vi "Draw Legend Cluster.vi"(8 "error in (no error)":errorcluster, 9 "Plot Area Ref":refnum<vi>, 10 "Number Of Rows":i32, 11 "2D Feather.lvclass in":refnum<class "2D Feather.lvclass">) -> (0 "error out":errorcluster, 1 "Legend Cluster":T1(array[cluster]), 3 "2D Feather.lvclass out":refnum<class "2D Feather.lvclass">)   [LabVIEW 2017, in "2D Feather.lvclass"]
uses:
  <vilib>/Math Plots/2D Math Plots/2D Feather/2D Feather/2D Feather.lvclass
  <vilib>/Math Plots/2D Math Plots/2D Feather/2D Feather/2D Feather.lvclass/2D Feather.ctl
  <vilib>/Math Plots/2D Math Plots/2D Plot/2D Plot/2D Plot.lvclass
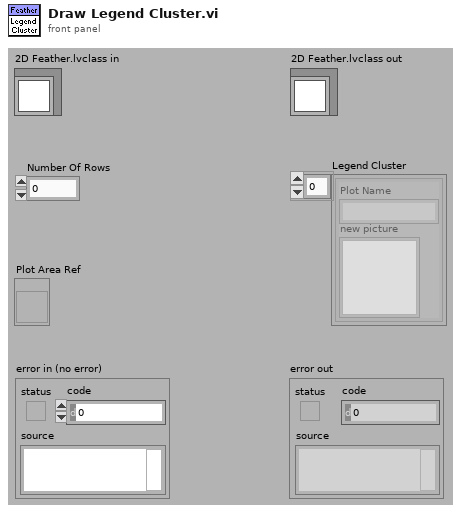
[diagram p1: front panel]
types:
  T1 = cluster{"Plot Name":string, "new picture":picture}[]
  T2 = typedef "2D Plot.lvclass/Plot Property Array.ctl" = T3[]
  T3 = typedef "2D Plot.lvclass/Plot Property.ctl" = cluster{"Bar Plot Style":u8, "DigitalLineStyle":u8, "TransitionLocation":u8, "Transition Type":u8, "Fill To":i16, "Fill/Pt. Color":u32, "Label Style":u8, "Line Style":u8, "Line Width":u8, "Plot Color":u32, "Plot Interpolation":u8, "Plot Name":string, "Point Style":u8, "Visible?":bool, "XScaleIdx":u32, "YScaleIdx":u32}
  T4 = cluster{"Width":u16, "Style":enum32{"Solid", "Dash", "Dot", "DashDot", "DashDotDot"}}
  T5 = cluster{"left":i16, "top":i16, "right":i16, "bottom":i16}
  T6 = cluster{"Plot Name":string, "new picture":picture}
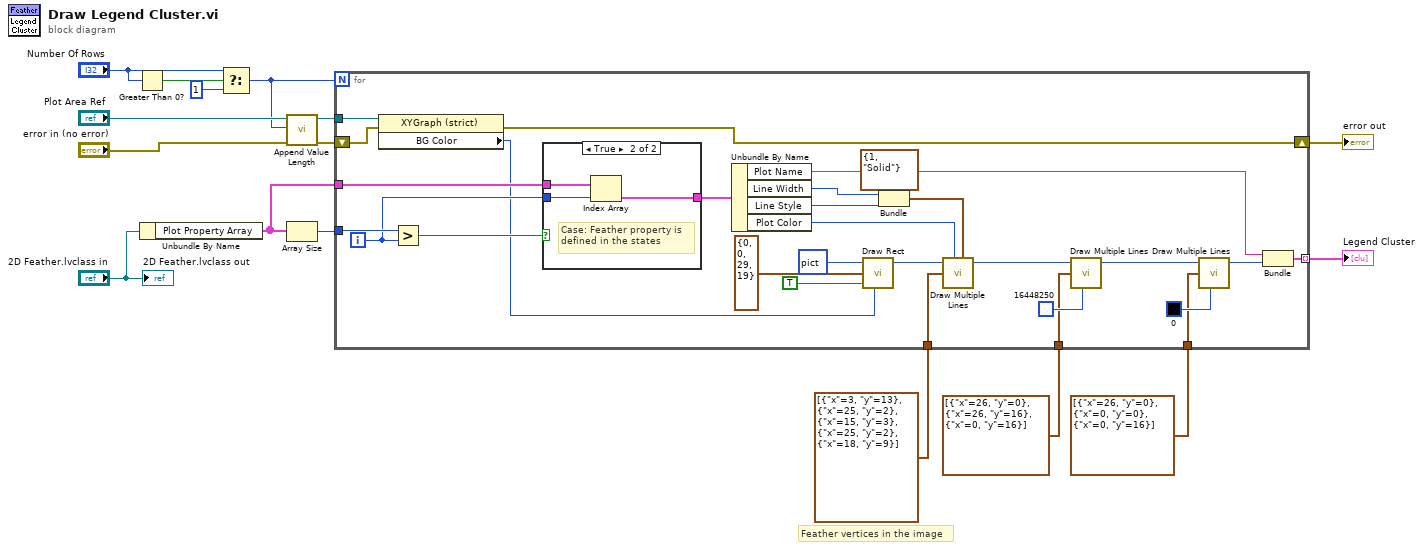
[diagram p0: block diagram]
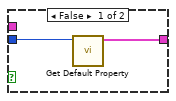
[diagram p2: hidden frame]
diagram:
  # "Feather vertices in the image"
  n1 = Greater Than 0?(x="Number Of Rows") -> (x > 0?=w16:bool)
  n2 = Unbundle By Name("2D Feather.lvclass in") -> ("Plot Property Array"=w13:T2)
  n3 = Select(t="Number Of Rows", s=w16, f=1) -> (s? t:f=w4:i32)
  n4 = call <vilib>:"Append Value Length.vi"("error in (no error)"="error in (no error)", "Expect Value Length"=w4, "Plot Area Ref In"="Plot Area Ref") -> ("error out"=w5:errorcluster, "Plot Area Ref Out"=w6:refnum<vi>)  [unwired: 1 in, 6 out]
  n5 = Array Size(array=w13) -> (size(s)=w14:i32)
  n6 = for {
    N: w4 -> [_]
    tunnel: w13 -> [w33]
    tunnel: [w37] -> w11 mode=indexing
    tunnel: w14 -> [w35]
    tunnel: w6 -> [w21]
    shift-right: [w17] -> w10
    shift-left: w5 -> [w22]
    tunnel: cluster{"x":i16, "y":i16}[] [{"x"=3, "y"=13}, {"x"=25, "y"=2}, {"x"=15, "y"=3}, {"x"=25, "y"=2}, {"x"=18, "y"=9}] ("line endpoints") -> [w20]
    tunnel: cluster{"x":i16, "y":i16}[] [{"x"=26, "y"=0}, {"x"=26, "y"=16}, {"x"=0, "y"=16}] ("line endpoints") -> [w19]
    tunnel: cluster{"x":i16, "y":i16}[] [{"x"=26, "y"=0}, {"x"=0, "y"=0}, {"x"=0, "y"=16}] ("line endpoints") -> [w18]
    i -> [w32]
    n7 = property class="XYGraph (strict)"(reference=w21, error in=w22) -> (error out=w17:errorcluster, "BG Color"=w23:u32)  [unwired: 1 out]
    n8 = Greater?(x=w35, y=w32) -> (0:w34:bool)
    n9 = case shown="True" w34 {
      tunnel: w33 -> [_ w49]
      tunnel: w32 -> [w45 w48]
      tunnel: [w46 w47] -> w31
      frame False {
        n10 = call <vilib>:"Get Default Property.vi"("Index"=w45) -> ("Temporary Property"=w46:T3)  [unwired: 3 in, 7 out]
      }
      frame True {
        # "Case: Feather property is \ndefined in the states"
        n11 = Index Array(array=w49, index=w48) -> (element=w47:T3)
      }
    }
    n12 = Unbundle By Name(w31) -> ("Plot Name"=w38:string, "Line Width"=w41:u8, "Line Style"=w40:u8, "Plot Color"=w30:u32)
    n13 = call <vilib>:"Draw Rect.vi"("picture"=picture data[5B], "rect"=T5 {"left"=0, "top"=0, "right"=29, "bottom"=19}, "fill?(F)"=TRUE, "color(black)"=w23) -> ("new picture"=w42:picture)  [unwired: 1 in, 4 out]
    n14 = Bundle(cluster=T4 {"Width"=1, "Style"=enum."Solid"} ("pen"), "Width"=w41, "Style"=w40) -> (w29:T4)
    n15 = call <vilib>:"Draw Multiple Lines.vi"("picture"=w42, "line endpoints"=w20, "color(black)"=w30, "pen"=w29) -> ("new picture"=w25:picture)  [unwired: 1 in, 4 out]
    n16 = call <vilib>:"Draw Multiple Lines.vi"("picture"=w25, "line endpoints"=w19, "color(black)"=u32 16448250) -> ("new picture"=w26:picture)  [unwired: 2 in, 4 out]
    n17 = call <vilib>:"Draw Multiple Lines.vi"("picture"=w26, "line endpoints"=w18, "color(black)"=u32 0) -> ("new picture"=w24:picture)  [unwired: 2 in, 4 out]
    n18 = Bundle("Plot Name"=w38, "new picture"=w24) -> (w37:T6)  [unwired: 1 out]
  }
  "Legend Cluster" <- w11
  "error out" <- w10
  "2D Feather.lvclass out" <- "2D Feather.lvclass in"
